vi "ADS1015_REG_CONFIG.vi"(0 "LINX Resource in":T2={"IO"=enum."Remote", "Interface"=enum."TCP", "LINX Device Config"={"Interface"=enum."TCP", "COM Port"="N/A", "TCP Configuration"={"IP Address"="panicattack", "Port"=6999}, "Device Family"=4, "Device ID"=1, "Device Name"="Raspberry Pi Model B", "TCP Ref"=refnum, "Channels"={"DI"=[2, 3, 4, 7, 8, 9, 10, 11, 14, 15, 17, 18, 22, 23, 24, 25, 27], "DO"=[2, 3, 4, 7, 8, 9, 10, 11, 14, 15, 17, 18, 22, 23, 24, 25, 27], "AI"=[], "AO"=[], "PWM"=[], "QE"=[], "UART"=[0], "I2C 2"=[0, 1], "SPI"=[0], "CAN"=[], "Servo"=[], "AI Ref (V)"=0.0, "AI Resolution (Bits)"=0, "AO Ref (V)"=0.0, "AO Resolution (Bits)"=0}}}, 3 "ADS1015 Reg Config":T8, 4 "I2C_Channel_platform":T1, 5 "Error In":errorcluster, 6 "I2C Slave Address (0)":u8) -> (14 "LINX Resource out":T2={"IO"=enum."Remote", "Interface"=enum."TCP", "LINX Device Config"={"Interface"=enum."TCP", "COM Port"="N/A", "TCP Configuration"={"IP Address"="panicattack", "Port"=6999}, "Device Family"=4, "Device ID"=1, "Device Name"="Raspberry Pi Model B", "TCP Ref"=refnum, "Channels"={"DI"=[2, 3, 4, 7, 8, 9, 10, 11, 14, 15, 17, 18, 22, 23, 24, 25, 27], "DO"=[2, 3, 4, 7, 8, 9, 10, 11, 14, 15, 17, 18, 22, 23, 24, 25, 27], "AI"=[], "AO"=[], "PWM"=[], "QE"=[], "UART"=[0], "I2C 2"=[0, 1], "SPI"=[0], "CAN"=[], "Servo"=[], "AI Ref (V)"=0.0, "AI Resolution (Bits)"=0, "AO Ref (V)"=0.0, "AO Resolution (Bits)"=0}}}, 19 "Error Out":errorcluster)   [LabVIEW 2014]
uses:
  <vilib>/MakerHub/LINX/Private/Type Defs/LINX Ref.ctl
  <vilib>/MakerHub/LINX/Private/Type Defs/Platform.ctl
  <vilib>/MakerHub/LINX/Private/Type Defs/Interface.ctl
  <vilib>/MakerHub/LINX/Private/Device/Type Defs/LINX Device Config.ctl
  <vilib>/MakerHub/LINX/Private/Device/Type Defs/TCP Config.ctl
  <vilib>/MakerHub/LINX/Private/Device/Type Defs/Channels.ctl
  User Defined/I2C_Platform_Selector.ctl
  <vilib>/MakerHub/LINX/Private/Local IO/LinxI2cWrite.vi
  <vilib>/MakerHub/LINX/Public/Utilities/Check Channel.vi
  <vilib>/MakerHub/LINX/Private/Local IO/Handle Errors.vi
  <vilib>/MakerHub/LINX/Private/Utilties/Generate Error.vi
  <vilib>/MakerHub/LINX/LMH-LINX.lvlib
  <vilib>/MakerHub/LINX/Private/Device/Device.lvlib
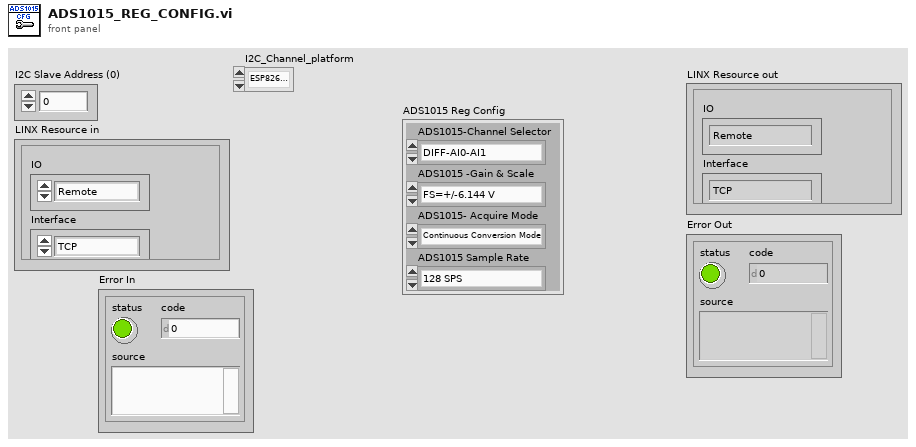
[diagram p1: front panel]
types:
  T1 = typedef "I2C_Platform_Selector.ctl" = enum16{"ESP8266-I2C", "Raspberry Pi-I2C"}
  T2 = typedef "LMH-LINX.lvlib/LINX Ref.ctl" = cluster{"IO":T3, "Interface":T4, "LINX Device Config":T5}
  T3 = typedef "LMH-LINX.lvlib/Platform.ctl" = enum16{"Remote", "Local"}
  T4 = typedef "LMH-LINX.lvlib/Interface.ctl" = enum16{"Serial", "TCP"}
  T5 = typedef "LMH-LINX.lvlib/Device.lvlib/LINX Device Config.ctl" = cluster{"Interface":T4, "COM Port":refnum<visa-resource-name>, "TCP Configuration":T6, "Device Family":u8, "Device ID":u8, "Device Name":string, "TCP Ref":refnum<k5>, "Channels":T7}
  T6 = typedef "LMH-LINX.lvlib/Device.lvlib/TCP Config.ctl" = cluster{"IP Address":string, "Port":u16}
  T7 = typedef "LMH-LINX.lvlib/Channels.ctl" = cluster{"DI":u8[], "DO":u8[], "AI":u8[], "AO":u8[], "PWM":u8[], "QE":u8[], "UART":u8[], "I2C 2":u8[], "SPI":u8[], "CAN":u8[], "Servo":u8[], "AI Ref (V)":dbl, "AI Resolution (Bits)":u8, "AO Ref (V)":dbl, "AO Resolution (Bits)":u8}
  T8 = cluster{"ADS1015-Channel Selector":enum8{"DIFF-AI0-AI1", "DIFF-AI0-AI3", "DIFF-AI1-AI3", "DIFF-AI2-AI3", "Single Ended - AI0", "Single Ended - AI1", "Single Ended - AI2", "Single Ended - AI3"}, "ADS1015 -Gain & Scale":enum8{"FS=+/-6.144 V", "FS=+/-4.096 V", "FS=+/-2.048 V", "FS=+/-1.024 V", "FS=+/-0.512 V", "FS=+/-0.256-A V", "FS=+/-0.256-B V", "FS=+/-0.256-C V"}, "ADS1015- Acquire Mode":enum16{"Continuous Conversion Mode", "Single Shot Mode"}, "ADS1015 Sample Rate":enum8{"128 SPS", "250 SPS", "490 SPS", "920 SPS", "1600 SPS", "2400 SPS", "3300 SPS", "3300 SPS A"}}
  T9 = enum8{"DIFF-AI0-AI1", "DIFF-AI0-AI3", "DIFF-AI1-AI3", "DIFF-AI2-AI3", "Single Ended - AI0", "Single Ended - AI1", "Single Ended - AI2", "Single Ended - AI3"}
  T10 = enum8{"FS=+/-6.144 V", "FS=+/-4.096 V", "FS=+/-2.048 V", "FS=+/-1.024 V", "FS=+/-0.512 V", "FS=+/-0.256-A V", "FS=+/-0.256-B V", "FS=+/-0.256-C V"}
  T11 = enum16{"Continuous Conversion Mode", "Single Shot Mode"}
  T12 = enum8{"128 SPS", "250 SPS", "490 SPS", "920 SPS", "1600 SPS", "2400 SPS", "3300 SPS", "3300 SPS A"}
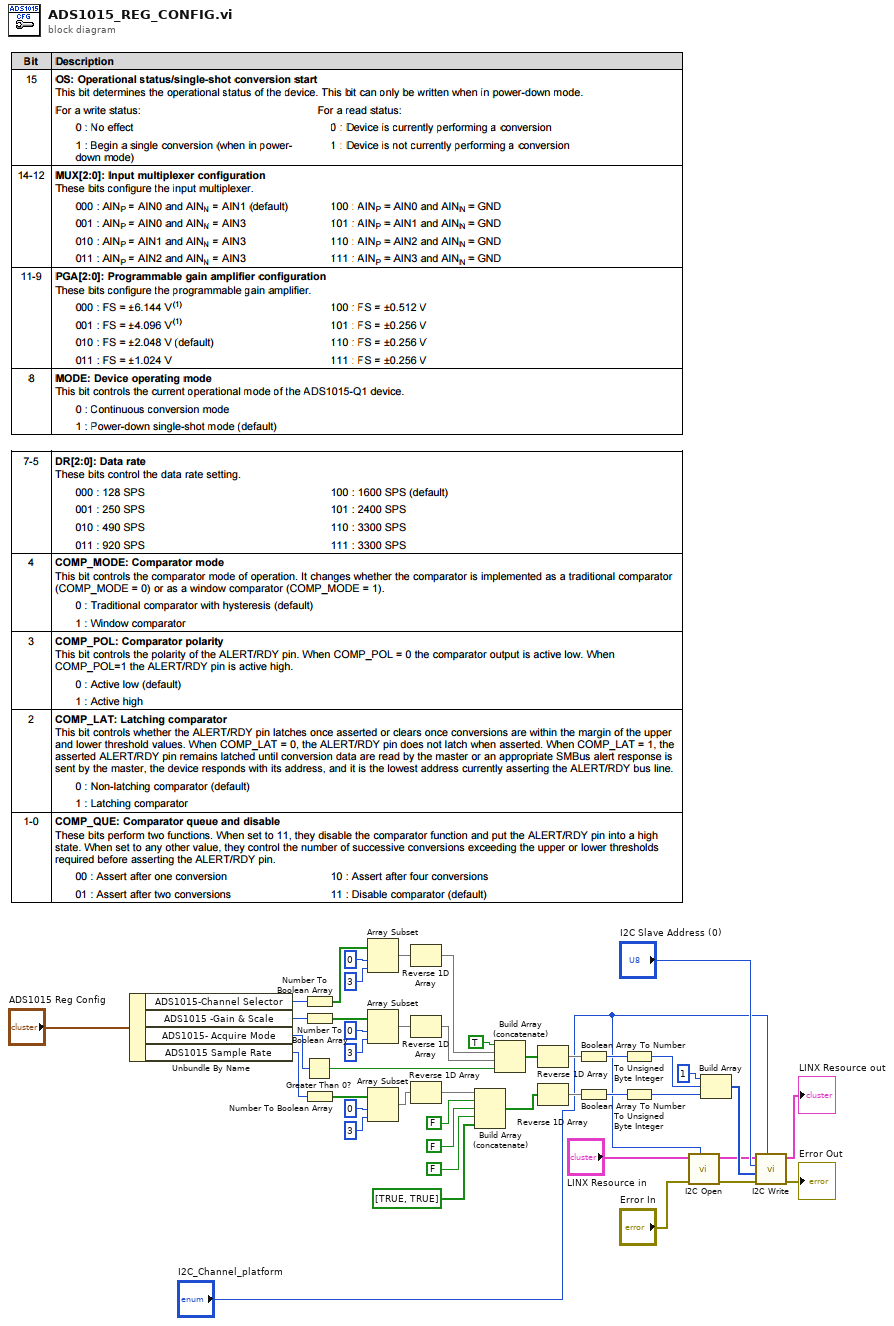
[diagram p0: block diagram]
diagram:
  n1 = Unbundle By Name("ADS1015 Reg Config") -> ("ADS1015-Channel Selector"=w13:T9, "ADS1015 -Gain & Scale"=w12:T10, "ADS1015- Acquire Mode"=w11:T11, "ADS1015 Sample Rate"=w10:T12)
  n2 = Greater Than 0?(x=w11) -> (x > 0?=w18:bool)
  n3 = Number To Boolean Array(number=w13) -> (Boolean array=w29:bool[])
  n4 = Number To Boolean Array(number=w12) -> (Boolean array=w21:bool[])
  n5 = Number To Boolean Array(number=w10) -> (Boolean array=w44:bool[])
  n6 = Array Subset(array=w29, index=0, length=3) -> (w26:bool[])
  n7 = Array Subset(array=w21, index=0, length=3) -> (w20:bool[])
  n8 = Array Subset(array=w44, index=0, length=3) -> (w41:bool[])
  n9 = Reverse 1D Array(array=w26) -> (reversed array=w24:bool[])
  n10 = Reverse 1D Array(array=w20) -> (reversed array=w19:bool[])
  n11 = Reverse 1D Array(array=w41) -> (reversed array=w40:bool[])
  n12 = Build Array (concatenate)(w40, FALSE, FALSE, FALSE, bool[] [TRUE, TRUE] ("array")) -> (w35:bool[])
  n13 = Build Array (concatenate)(TRUE, w24, w19, w18) -> (w17:bool[])
  n14 = Reverse 1D Array(array=w17) -> (reversed array=w16:bool[])
  n15 = Reverse 1D Array(array=w35) -> (reversed array=w34:bool[])
  n16 = Boolean Array To Number(Boolean array=w16) -> (number=w15:u32)
  n17 = Boolean Array To Number(Boolean array=w34) -> (number=w33:u32)
  n18 = To Unsigned Byte Integer(number=w15) -> (unsigned 8bit integer=w32:u8)
  n19 = To Unsigned Byte Integer(number=w33) -> (unsigned 8bit integer=w30:u8)
  n20 = call <vilib>:"I2C Open.vi"("I2C Channel (0)"="I2C_Channel_platform", "Error In"="Error In", "LINX Resource"="LINX Resource in") -> ("Error Out"=w3:errorcluster, "LINX Resource"=w4:T2)  [unwired: 7 in]
  n21 = Build Array(u8 1 ("element"), w32, w30) -> (w9:u8[])
  n22 = call <vilib>:"I2C Write.vi"("I2C Channel"="I2C_Channel_platform", "Error In"=w3, "Data"=w9, "I2C Slave Address (0)"="I2C Slave Address (0)", "LINX Resource"=w4) -> ("Error Out"=→"Error Out":errorcluster, "LINX Resource"=→"LINX Resource out":T2)  [unwired: 5 in]
